vi "MEMR-Compute Metrics (NF).vi"(0 "Gain spectra in":cluster{"Freq (Hz)":dbl[], "Mag":dbl[]}[](array[cluster]), 5 "Compute":enum16{"Mean", "Sum"}(ring), 7 "Scale":enum16{"Linear", "Log"}(ring), 9 "Fpeak":dbl[](array[numeric]), 11 "Measure":T1(ring)) -> (4 "Gain spectra out":cluster{"Freq (Hz)":dbl[], "Mag":dbl[]}[](array[cluster]), 8 "Metrics":dbl[](array[numeric]))   [LabVIEW 2020]
uses:
  <vilib>/Analysis/baseanly.llb/Mean (DBL).vi
  Utility VIs/Array Manipulation VIs/Irregular Array Subset (DBL).vi
  Utility VIs/Math VIs/interp1 (1D).vi
  Utility VIs/Math VIs/dB to Linear (1D).vi
  Utility VIs/Math VIs/Linear to dB (scalar).vi
  <vilib>/Analysis/NI_AALBase.lvlib
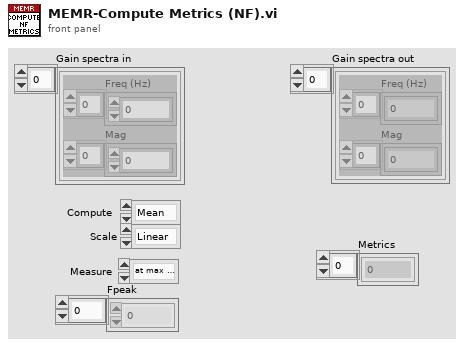
[diagram p1: front panel]
types:
  T1 = enum16{"at max mag", "at max gain", "over window", "optimize", "Keefe"}
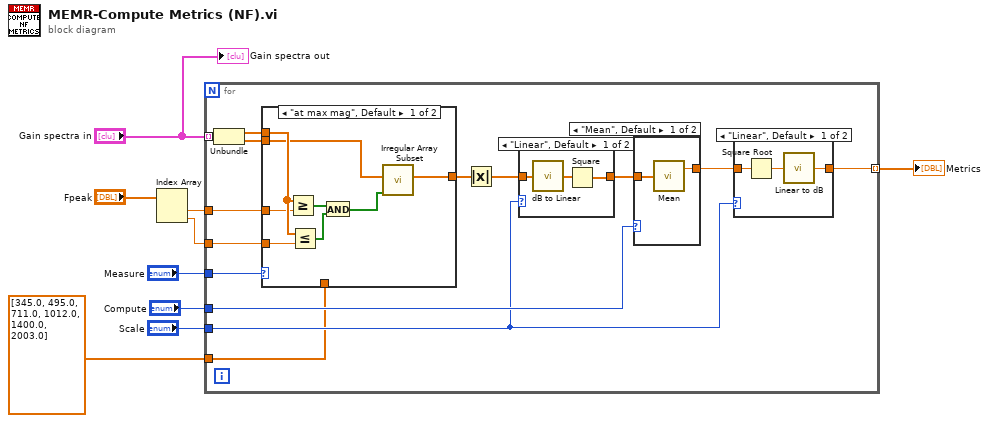
[diagram p0: block diagram]
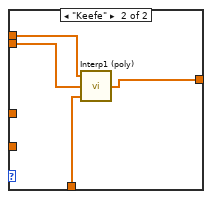
[diagram p2: hidden frame]
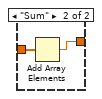
[diagram p3: hidden frame]
diagram:
  n1 = Index Array(array="Fpeak") -> (element #1=w6:dbl, element #2=w5:dbl)  [unwired: 2 in]
  n2 = for {
    tunnel: "Gain spectra in" -> [w23] mode=indexing
    tunnel: [w12] -> w8 mode=indexing
    tunnel: w6 -> [w21]
    tunnel: w5 -> [w20]
    tunnel: "Compute" -> [w14]
    tunnel: "Scale" -> [w13]
    tunnel: "Measure" -> [w11]
    tunnel: dbl[] [345.0, 495.0, 711.0, 1012.0, 1400.0, 2003.0] -> [w10]
    n3 = Unbundle(w23) -> ("Freq (Hz)"=w22:dbl[], "Mag"=w15:dbl[])
    n4 = case shown="\"at max mag\", Default" w11 {
      tunnel: w22 -> [w29 w35]
      tunnel: w21 -> [w28 _]
      tunnel: w20 -> [w27 _]
      tunnel: [w26 w32] -> w16
      tunnel: w15 -> [w25 w34]
      tunnel: w10 -> [_ w33]
      frame "at max mag", Default {
        n5 = Greater Or Equal?(x=w29, y=w28) -> (x >= y?=w30:bool[])
        n6 = Less Or Equal?(x=w29, y=w27) -> (x <= y?=w31:bool[])
        n7 = And(x=w30, y=w31) -> (x .and. y?=w24:bool[])
        n8 = call-poly "Irregular Array Subset.vi"("Mask"=w24, "Array"=w25) -> ("Array Subset"=w26:dbl[])  [unwired: 8 in, 1 out]
      }
      frame "Keefe" {
        n9 = call-poly "Interp1 (poly).vi"("X"=w35, "Y"=w34, "U"=w33) -> ("V"=w32:dbl[])  [unwired: 2 in]
      }
    }
    n10 = Absolute Value(x=w16) -> (abs(x)=w19:dbl[])
    n11 = case shown="\"Linear\", Default" w13 {
      tunnel: [w42 w43] -> w18
      tunnel: w19 -> [w41 w43]
      frame "Linear", Default {
        n12 = call-poly "dB to Linear.vi"("dB"=w41) -> ("linear"=w40:dbl[])
        n13 = Square(x=w40) -> (x^2=w42:dbl[])
      }
      frame "Log" {
      }
    }
    n14 = case shown="\"Mean\", Default" w14 {
      tunnel: [w37 w39] -> w17
      tunnel: w18 -> [w36 w38]
      frame "Mean", Default {
        n15 = call-poly <vilib>:"Mean.vi"("X"=w36) -> ("mean"=w37:dbl)  [unwired: 1 out]
      }
      frame "Sum" {
        n16 = Add Array Elements(numeric array=w38) -> (sum=w39:dbl)
      }
    }
    n17 = case shown="\"Linear\", Default" w13 {
      tunnel: [w46 w47] -> w12
      tunnel: w17 -> [w44 w47]
      frame "Linear", Default {
        n18 = Square Root(x=w44) -> (sqrt(x)=w45:dbl)
        n19 = call-poly "Linear to dB.vi"("Linear"=w45) -> ("dB"=w46:dbl)
      }
      frame "Log" {
      }
    }
  }
  "Metrics" <- w8
  "Gain spectra out" <- "Gain spectra in"
